vi "init data structures.vi"(8 "error in":errorcluster, 9 "data allocations":T1, 10 "shared memory configuration":refnum<class "Shared Memory configuration.lvclass">, 11 "shared memory runtime in":refnum<class "Shared Memory runtime.lvclass">) -> (0 "error out":errorcluster, 3 "shared memory runtime out":refnum<class "Shared Memory runtime.lvclass">)   [LabVIEW 2014, in "Shared Memory runtime.lvclass"]
uses:
  Shared Memory runtime.lvclass
  configuration/Shared Memory configuration.lvclass
  <vilib>/NI/Tag Bus Module Framework/channel/data tables.ctl
  <vilib>/NI/Tag Bus/dictionary/data dictionary.lvclass
  <vilib>/NI/Tag Bus/dictionary table pair.ctl
  <vilib>/NI/Tag Bus/table/data table.ctl
  <vilib>/NI/Tag Bus Module Framework/channel/TBM channel.lvclass/TBM channel.ctl
  <vilib>/NI/Tag Bus Module Framework/channel/TBM channel.lvclass
  <vilib>/NI/Tag Bus/table/data table.lvlib
  <vilib>/NI/Tag Bus/tag bus.lvlib
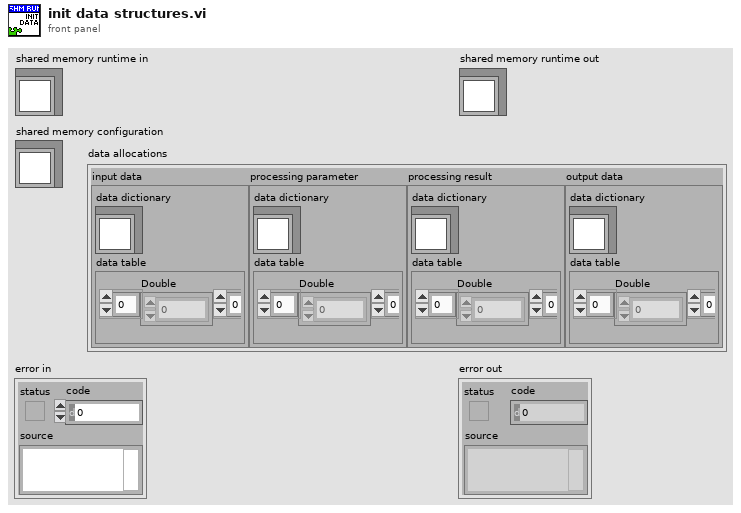
[diagram p1: front panel]
types:
  T1 = typedef "TBM channel.lvclass/data tables.ctl" = cluster{"input data":T2, "processing parameter":T2, "processing result":T2, "output data":T2}
  T2 = typedef "tag bus.lvlib/dictionary table pair.ctl" = cluster{"data dictionary":refnum<class "data dictionary.lvclass">, "data table":T3}
  T3 = typedef "tag bus.lvlib/data table.lvlib/data table.ctl" = cluster{"Double":dbl[], "Single":sgl[], "I64":i64[], "I32":i32[], "I16":i16[], "I8":i8[], "U64":u64[], "U32":u32[], "U16":u16[], "U8":u8[], "Boolean":bool[], "String":string[], "Array of Double":cluster{"DBL Array":dbl[]}[], "Array of Single":cluster{"SGL Array":sgl[]}[], "Array of I64":cluster{"I64 Array":i64[]}[], "Array of I32":cluster{"I32 Array":i32[]}[], "Array of I16":cluster{"I16 Array":i16[]}[], "Array of I8":cluster{"I8 Array":i8[]}[], "Array of U64":cluster{"U64 Array":u64[]}[], "Array of U32":cluster{"U32 Array":u32[]}[], "Array of U16":cluster{"U16 Array":u16[]}[], "Array of U8":cluster{"U8 Array":u8[]}[], "Array of Boolean":cluster{"Boolean Array":bool[]}[], "Array of String":cluster{"String Array":string[]}[]}
  T4 = typedef "Shared Memory configuration.lvclass/Memory Allocation.ctl" = cluster{"shared memory name":string, "Lines":T5[]}
  T5 = typedef "Shared Memory configuration.lvclass/Line.ctl" = cluster{"channel":refnum<class "TBM channel.lvclass">}
  T6 = typedef "TBM channel.lvclass/channel classification.ctl" = enum16{"input data", "output data", "processing parameter", "processing result"}
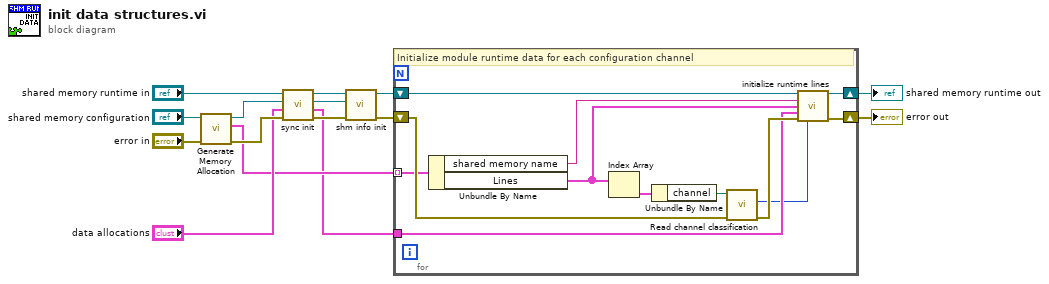
[diagram p0: block diagram]
diagram:
  n1 = call "Generate Memory Allocation.vi"("error in"="error in", "Shared Memory configuration in"="shared memory configuration") -> ("error out"=w12:errorcluster, "Memory Allocations"=w8:T4[], "Shared Memory configuration out"=w1:refnum<class "Shared Memory configuration.lvclass">)  [unwired: 7 in]
  n2 = call "sync init.vi"("error in (no error)"=w12, "data allocations in"="data allocations", "shared memory configuration in"=w1, "shared memory runtime in"="shared memory runtime in") -> ("error out"=w4:errorcluster, "data allocations out"=w2:T1, "shared memory configuration out"=w5:refnum<class "Shared Memory configuration.lvclass">, "shared memory runtime out"=w7:refnum<class "Shared Memory runtime.lvclass">)  [unwired: 4 in]
  n3 = call "shm info init.vi"("error in (no error)"=w4, "shared memory configuration in"=w5, "shared memory runtime in"=w7) -> ("error out"=w3:errorcluster, "shared memory runtime out"=w6:refnum<class "Shared Memory runtime.lvclass">)  [unwired: 6 in, 1 out]
  n4 = for {
    tunnel: w2 -> [w22]
    shift-right: [w17] -> w15
    shift-left: w6 -> [w21]
    shift-right: [w16] -> w14
    shift-left: w3 -> [w27]
    tunnel: w8 -> [w26] mode=indexing
    # "Initialize module runtime data for each configuration channel"
    n5 = Unbundle By Name(w26) -> ("shared memory name"=w18:string, "Lines"=w19:T5[])
    n6 = Index Array(array=w19) -> (element=w25:T5)  [unwired: 1 in]
    n7 = Unbundle By Name(w25) -> ("channel"=w24:refnum<class "TBM channel.lvclass">)
    n8 = call <vilib>:"Read channel classification.vi"("error in"=w27, "channel in"=w24) -> ("error out"=w23:errorcluster, "channel classification"=w20:T6)  [unwired: 7 in, 1 out]
    n9 = call "initialize runtime lines.vi"("Shared Memory runtime in"=w21, "shared memory name"=w18, "Lines"=w19, "data allocations in"=w22, "error in (no error)"=w23, "channel classification"=w20) -> ("Shared Memory runtime out"=w17:refnum<class "Shared Memory runtime.lvclass">, "error out"=w16:errorcluster)  [unwired: 8 in]
  }
  "error out" <- w14
  "shared memory runtime out" <- w15
